vi "Init Msg Output.vi"() -> (2 "Msg Output":refnum<class "Msg Output.lvclass">)   [LabVIEW 2020, in "jettl.lvlib" / "Start jettl Msg.lvlib" / "Start Msg Output.lvlib"]
doc: "jettl 6.14.1.98\nNathan Davis - Nathan Davis\nCopyright (c) 2026, Nathan Davis\nMIT"
uses:
  Start Msg Output.lvlib
  Msg Output/Msg Output.lvclass
  Start Msg Output/Start Msg Output.lvclass
  C:/git/jettl/src/jettl/jettl/Msg Output/Msg Output.lvclass
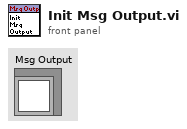
[diagram p1: front panel]
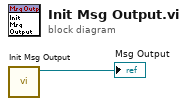
[diagram p0: block diagram]
diagram:
  n1 = call "Init Msg Output.vi"() -> ("Start Msg Output out"=→"Msg Output":refnum<class "Start Msg Output.lvclass">)  [unwired: 11 in]
